vi "Wait with error passthrough.vi"(10 "error in":errorcluster, 11 "milliseconds to wait":u32) -> (2 "error out":errorcluster)   [LabVIEW 2016]
doc: "The built-in Wait function is awkward for the data flow model because it has only one input. This simply makes it wait for an error input before executing. Therefore, no sequence structure is necessary."
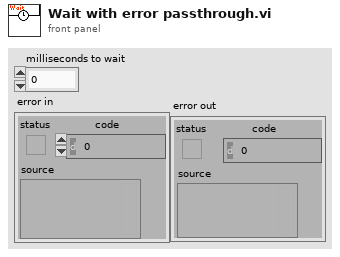
[diagram p1: front panel]
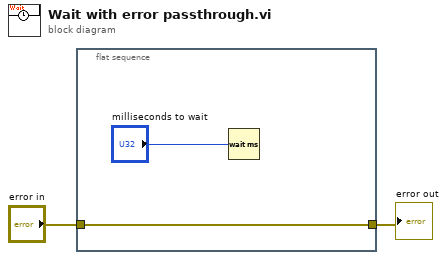
[diagram p0: block diagram]
diagram:
  n1 = flat-sequence {
    tunnel: "error in" -> [w3]
    tunnel: [w3] -> w1
    frame #0 {
      n2 = Wait (ms)(milliseconds to wait="milliseconds to wait") -> ()  [unwired: 1 out]
    }
  }
  "error out" <- w1
